vi "get enum strings.vi"(8 "error in":errorcluster, 11 "displayable in":refnum<class "displayable.lvclass">) -> (0 "error out":errorcluster, 2 "Enum Names":string[](array[string]), 3 "displayable out":refnum<class "displayable.lvclass">)   [LabVIEW 2013, in "displayable.lvclass"]
uses:
  displayable.lvclass
  <vilib>/Utility/VariantDataType/VariantType.lvlib
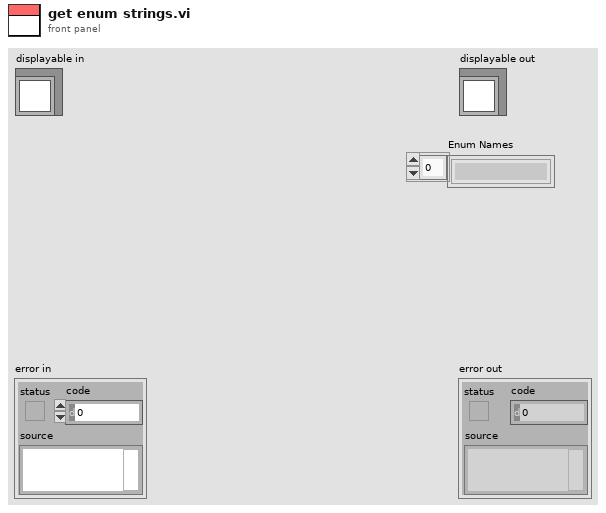
[diagram p1: front panel]
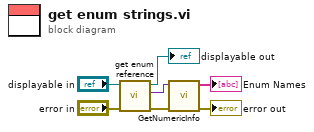
[diagram p0: block diagram]
diagram:
  n1 = call-dynamic "get enum reference.vi"("error in"="error in", "displayable in"="displayable in") -> ("error out"=w4:errorcluster, "enum"=w3:variant, "displayable out"=→"displayable out":refnum<class "displayable.lvclass">)  [unwired: 7 in]
  n2 = call <vilib>:"GetNumericInfo.vi"("error in (no error)"=w4, "Variant"=w3) -> ("error out"=→"error out":errorcluster, "EnumNames"=→"Enum Names":string[])  [unwired: 6 in, 2 out]
